vi "Unflatten-MouseMotionEvent.vi"(8 "error in (no error)":errorcluster, 11 "Event Binary Data":string) -> (0 "error out":errorcluster, 3 "MouseMotionEvent":T1 {"state" items=["SDL_BUTTON_LEFT"=1, "SDL_BUTTON_MIDDLE"=2, "SDL_BUTTON_RIGHT"=3, "SDL_BUTTON_X1"=4, "SDL_BUTTON_X2"=5]})   [LabVIEW 2024, in "SDL3.lvlib" / "Events.lvlib"]
uses:
  Events.lvlib
  Video/WindowID--integer.ctl
  Video/Video.lvlib
  Mouse/MouseID--integer.ctl
  Mouse/Mouse.lvlib
  Mouse/MouseButtonFlags--ring.ctl
  MouseMotionEvent--cluster.ctl
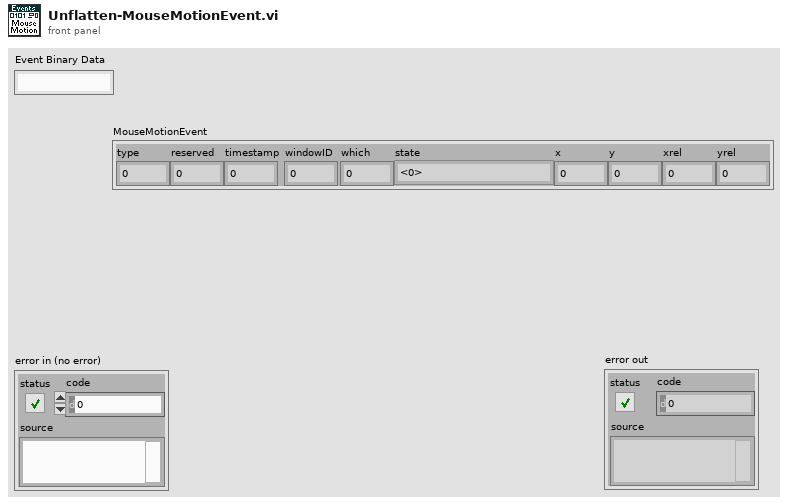
[diagram p1: front panel]
types:
  T1 = typedef "SDL3.lvlib/Events.lvlib/MouseMotionEvent--cluster.ctl" = cluster{"type":u32, "reserved":u32, "timestamp":u64, "windowID":T2, "which":T3, "state":T4, "x":sgl, "y":sgl, "xrel":sgl, "yrel":sgl}
  T2 = typedef "SDL3.lvlib/Video.lvlib/WindowID--integer.ctl" = u32
  T3 = typedef "SDL3.lvlib/Mouse.lvlib/MouseID--integer.ctl" = u32
  T4 = typedef "SDL3.lvlib/Mouse.lvlib/MouseButtonFlags--ring.ctl" = u32
  T5 = cluster{"type":u32, "reserved":u32, "timestamp":u64, "windowID":T2, "which":T3, "state":T4, "x":sgl, "y":sgl, "xrel":sgl, "yrel":sgl}
  T6 = enum16{"big-endian, network order", "native, host order", "little-endian"}
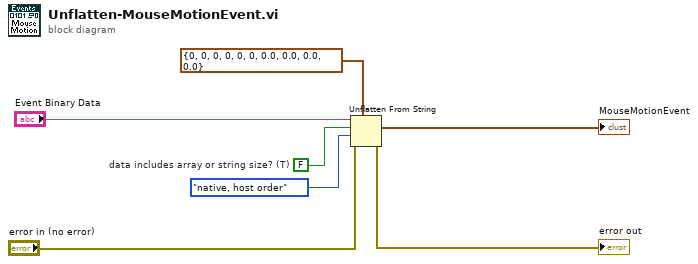
[diagram p0: block diagram]
diagram:
  w3 = FALSE  # data includes array or string size? (T)
  n1 = Unflatten From String(type=T5 {"type"=0, "reserved"=0, "timestamp"=0, "windowID"=0, "which"=0, "state"=0, "x"=0.0, "y"=0.0, "xrel"=0.0, "yrel"=0.0} ("MouseMotionEvent"), binary string="Event Binary Data", data includes array or string size? (T)=w3, byte order (0:big-endian, network order)=T6."native, host order", error in (no error)="error in (no error)") -> (value=→"MouseMotionEvent":T5, error out=→"error out":errorcluster)  [unwired: 1 out]
